vi "tm_getarea_42_ma.vi"(8 "error in (no error)":errorcluster, 11 "Handle in":u32) -> (0 "error out":errorcluster, 1 "V Offset":T1, 2 "H Offset":T1, 3 "Handle out":u32, 4 "H Width":T1, 6 "V Width":T1)   [LabVIEW 2023]
uses:
  tmcamcon.dll
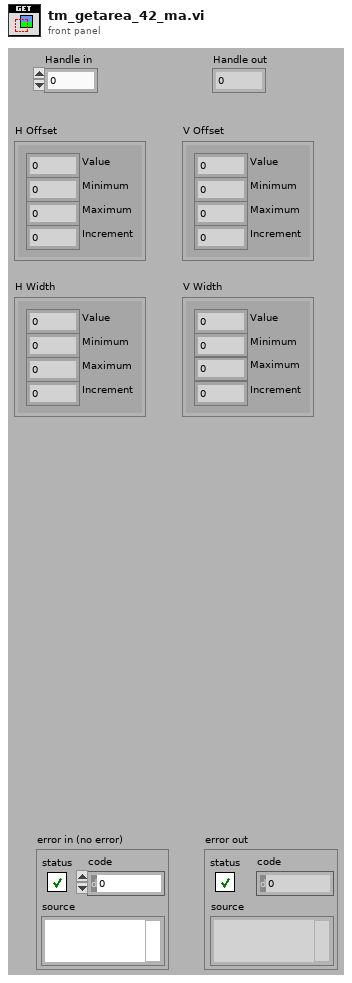
[diagram p1: front panel]
types:
  T1 = cluster{"Value":i32, "Minimum":i32, "Maximum":i32, "Increment":i32}
  T2 = cluster{"hov":i32, "hon":i32, "hox":i32, "hoi":i32}
  T3 = cluster{"hwv":i32, "hwn":i32, "hwx":i32, "hwi":i32}
  T4 = cluster{"vov":i32, "von":i32, "vox":i32, "voi":i32}
  T5 = cluster{"vwv":i32, "vwn":i32, "vwx":i32, "vwi":i32}
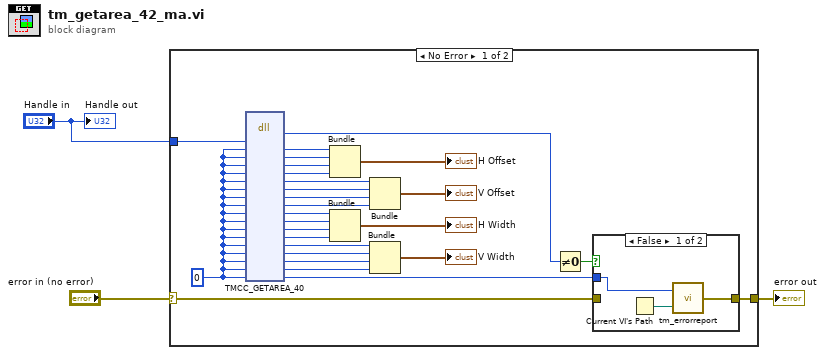
[diagram p0: block diagram]
diagram:
  n1 = case shown="No Error" "error in (no error)" {
    selector: "error in (no error)" -> [w15 w35]
    tunnel: [w12 w35] -> w2
    tunnel: "Handle in" -> [w16 _]
    frame No Error {
      w26 = 0
      n2 = dll-call lib="tmcamcon.dll" fn="TMCC_GETAREA_40"("index"=w16, "hov"=w26, "hon"=w26, "hox"=w26, "hoi"=w26, "vov"=w26, "von"=w26, "vox"=w26, "voi"=w26, "hwv"=w26, "hwn"=w26, "hwx"=w26, "hwi"=w26, "vwv"=w26, "vwn"=w26, "vwx"=w26, "vwi"=w26, "Erval"=w26) -> ("return type"=w30:u32, "hov"=w11:i32, "hon"=w28:i32, "hox"=w29:i32, "hoi"=w27:i32, "vov"=w9:i32, "von"=w25:i32, "vox"=w24:i32, "voi"=w23:i32, "hwv"=w7:i32, "hwn"=w22:i32, "hwx"=w21:i32, "hwi"=w20:i32, "vwv"=w5:i32, "vwn"=w19:i32, "vwx"=w18:i32, "vwi"=w17:i32, "Erval"=w13:i32)  [unwired: 4 in, 2 out]
      n3 = Bundle("hov"=w11, "hon"=w28, "hox"=w29, "hoi"=w27) -> (→"H Offset":T2)  [unwired: 1 in]
      n4 = Bundle("hwv"=w7, "hwn"=w22, "hwx"=w21, "hwi"=w20) -> (→"H Width":T3)  [unwired: 1 in]
      n5 = Bundle("vov"=w9, "von"=w25, "vox"=w24, "voi"=w23) -> (→"V Offset":T4)  [unwired: 1 in]
      n6 = Bundle("vwv"=w5, "vwn"=w19, "vwx"=w18, "vwi"=w17) -> (→"V Width":T5)  [unwired: 1 in]
      n7 = Not Equal To 0?(x=w30) -> (x != 0?=w14:bool)
      n8 = case shown="False" w14 {
        tunnel: w15 -> [_ w34]
        tunnel: [w32 w34] -> w12
        tunnel: w13 -> [w31 _]
        frame False {
          n9 = Current VI's Path() -> (path=w33:path)
          n10 = call "tm_errorreport.vi"("Source"=w33, "Error"=w31) -> ("error out"=w32:errorcluster)
        }
        frame True {
        }
      }
    }
    frame Error {
    }
  }
  "error out" <- w2
  "Handle out" <- "Handle in"
